vi "Write Message.vi"(8 "error in (no error)":errorcluster, 10 "Message":string, 11 "CLILogger in":refnum<class "CLILogger.lvclass">) -> (0 "error out":errorcluster, 3 "CLILogger out":refnum<class "CLILogger.lvclass">)   [LabVIEW 2020, in "GPackTools.lvlib" / "CLILogger.lvclass"]
uses:
  CLILogger.lvclass
  Log Entry.ctl
  CLILogger.lvclass/CLILogger.ctl
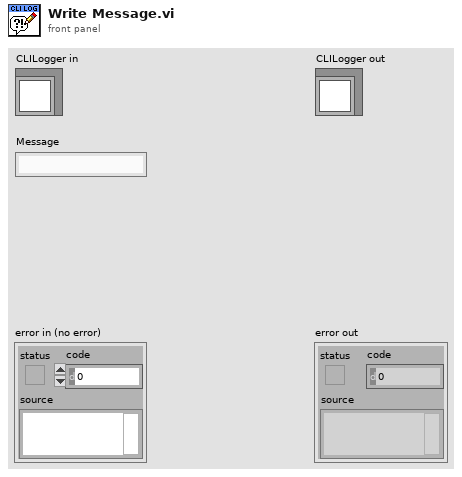
[diagram p1: front panel]
types:
  T1 = typedef "GPackTools.lvlib/CLILogger.lvclass/Log Entry.ctl" = cluster{"Time Stamp":timestamp, "Message":string}
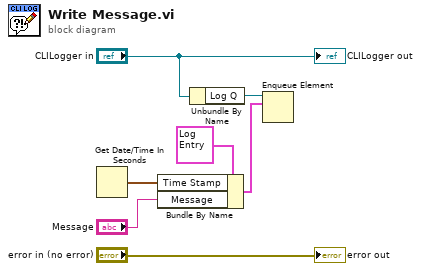
[diagram p0: block diagram]
diagram:
  n1 = Get Date/Time In Seconds() -> (seconds since 1Jan1904=w1:timestamp)
  n2 = Bundle By Name(cluster=T1 {"Time Stamp"=timestamp(0 s since 1904-01-01), "Message"=""} ("Log Entry"), "Time Stamp"=w1, "Message"="Message") -> (w3:T1)
  n3 = Unbundle By Name("CLILogger in") -> ("Log Q"=w4:refnum<queue>)
  n4 = Enqueue Element(queue=w4, element=w3) -> ()  [unwired: 2 in, 3 out]
  "error out" <- "error in (no error)"
  "CLILogger out" <- "CLILogger in"
